vi "C4Dev_getFeatureList.vi"(0 "c4dev in":refnum<k24>, 11 "error in":errorcluster) -> (4 "c4dev out":refnum<k24>, 6 "c4ftrs out":refnum<k24>[](array[refnum]), 15 "error out":errorcluster)   [LabVIEW 2015, in "libC4HdlLV.lvlib"]
uses:
  libC4HdlLV.lvlib
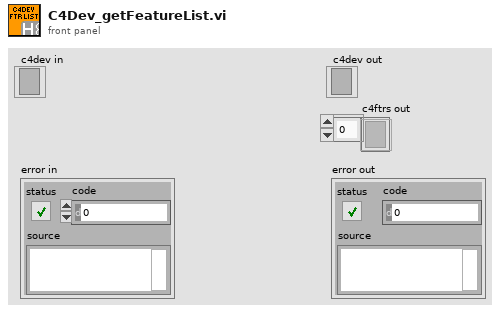
[diagram p1: front panel]
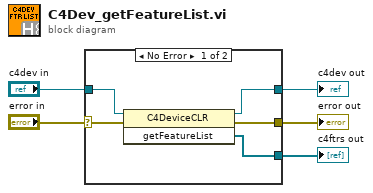
[diagram p0: block diagram]
diagram:
  n1 = case shown="No Error" "error in" {
    selector: "error in" -> [w7 w12]
    tunnel: [w6 w12] -> w4
    tunnel: "c4dev in" -> [w10 w11]
    tunnel: [w8 w11] -> w2
    tunnel: [w9 _] -> w1
    frame No Error {
      n2 = invoke class="C4DeviceCLR" method="getFeatureList"(reference=w10, error in=w7) -> (reference out=w8:refnum<k24>, error out=w6:errorcluster, "getFeatureList"=w9:refnum<k24>[])  [unwired: 1 in]
    }
    frame Error {
    }
  }
  "error out" <- w4
  "c4dev out" <- w2
  "c4ftrs out" <- w1
